vi "Exe1.vi"() -> ()   [LabVIEW 2017]
uses:
  <vilib>/Analysis/4window.llb/windowTd.ctl
  <vilib>/sound2/lvsound2.llb/Sound Data Format.ctl
  <vilib>/sound2/lvsound2.llb/Sampling Mode.ctl
  <extravilib>/ChannelInstances/Stream-a[.](wfm(dbl))/Read With Abort.vi
  <extravilib>/ChannelInstances/Stream-a[.](wfm(dbl))/Write With Abort.vi
  <extravilib>/ChannelInstances/Stream-a[.](wfm(dbl))/EndpointRead.vi
  <extravilib>/ChannelInstances/Stream-a[.](wfm(dbl))/Endpoint.vi
  <extravilib>/ChannelInstances/Stream-a[.](wfm(dbl))/Instantiate.vi
  <extravilib>/ChannelInstances/Stream-a[.](wfm(dbl))/)Channel.vi
  <resource>/ChannelSupport/_ChannelSupport/WaitIfNeeded.vi
  <vilib>/Waveform/WDTFileIO.llb/Export Waveforms To Spreadsheet File (1D).vi
  <vilib>/measure/maspectr.llb/FFT Power Spectrum and PSD for N Chan.vi
  <vilib>/sound2/lvsound2.llb/Sound Input Read (DBL).vi
  <extravilib>/ChannelInstances/Stream-a[.](wfm(dbl)).lvlib
  <vilib>/measure/NI_MAPro.lvlib
  <vilib>/Analysis/NI_AALPro.lvlib
panel:
  in  "file path":path=path "C:/Polimi/2020-data-acquisition-systems/04-ExamPreparation/data.txt"
  out "Acquired Audio PSD":cluster{"f0":dbl, "df":dbl, "magnitude":dbl[]}[](graph)
  in  "dB On (F)":bool
  in  "window":T1=1 items=["Rectangle"=0, "Hanning"=1, "Hamming"=2, "Blackman-Harris"=3, "Exact Blackman"=4, "Blackman"=5, "Flat Top"=6, "4 Term B-Harris "=7, "7 Term B-Harris"=8, "Low Sidelobe"=9, "Blackman Nuttall"=11, "Triangle"=30, "Bartlett-Hanning"=31, "Bohman"=32, "Parzen"=33, "Welch"=34, "Kaiser"=60, "Dolph-Chebyshev"=61, "Gaussian"=62]
  out "Positive Peak":dbl
  out "Negative Peak":dbl
  out "Mean (DC)":dbl
  out "Acquired Audio":waveform(dbl)[](graph)
  in  "stop":bool
  # "Exercise 1"
  # "Exercise 2"
  # "Exercise 3"
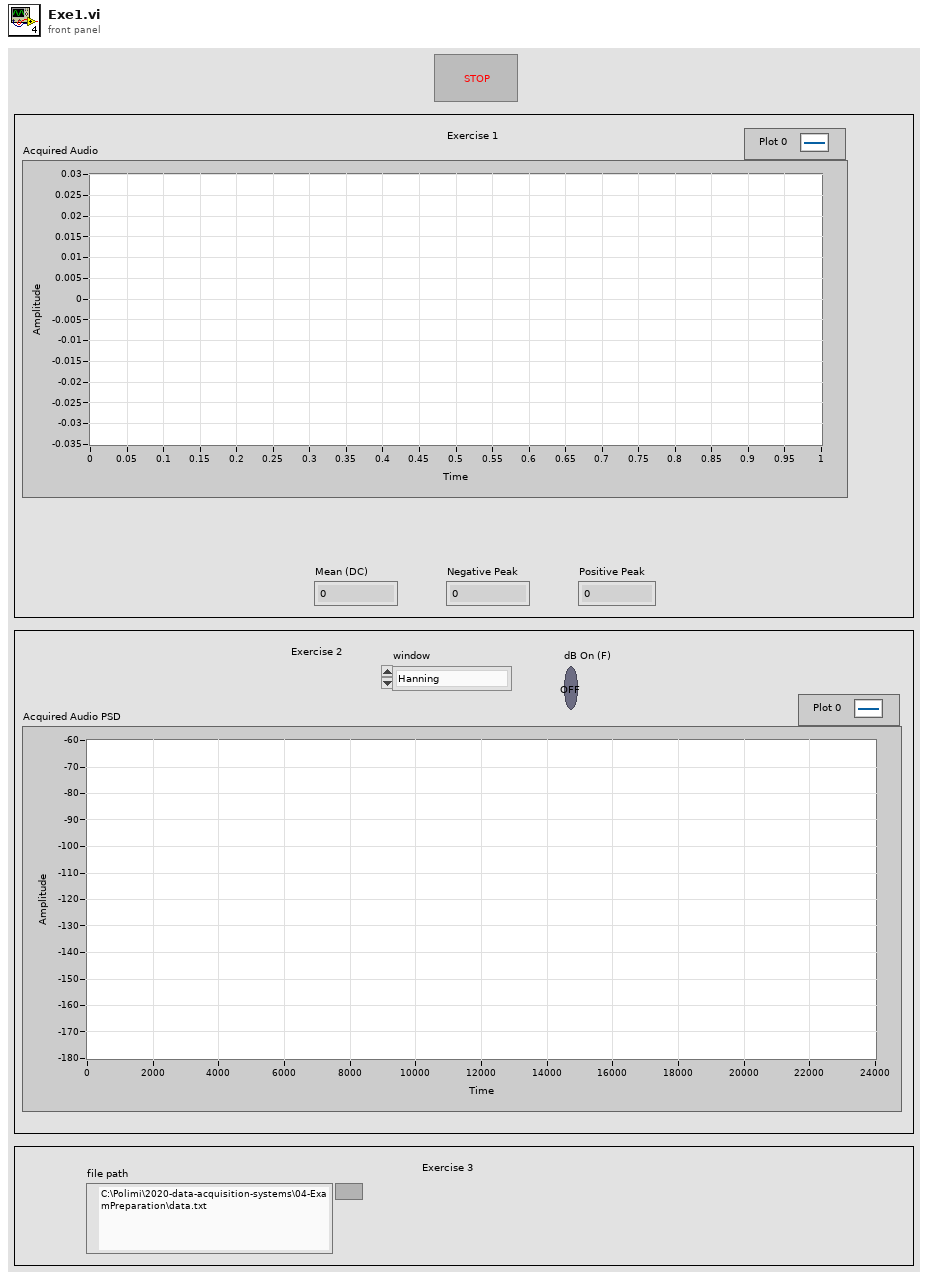
[diagram p1: front panel]
types:
  T1 = typedef "NI_AALPro.lvlib/windowTd.ctl" = u32
  T2 = typedef "Sampling Mode.ctl" = i32
  T3 = typedef "Sound Data Format.ctl" = cluster{"sample rate (S/s)":dbl, "number of channels":i32, "bits per sample":i32}
  T4 = typedef "Sound Input Task ID.ctl" = u32
  T5 = typedef "Stream-a[.](wfm(dbl)).lvlib/)Channel.ctl" = refnum<queue>
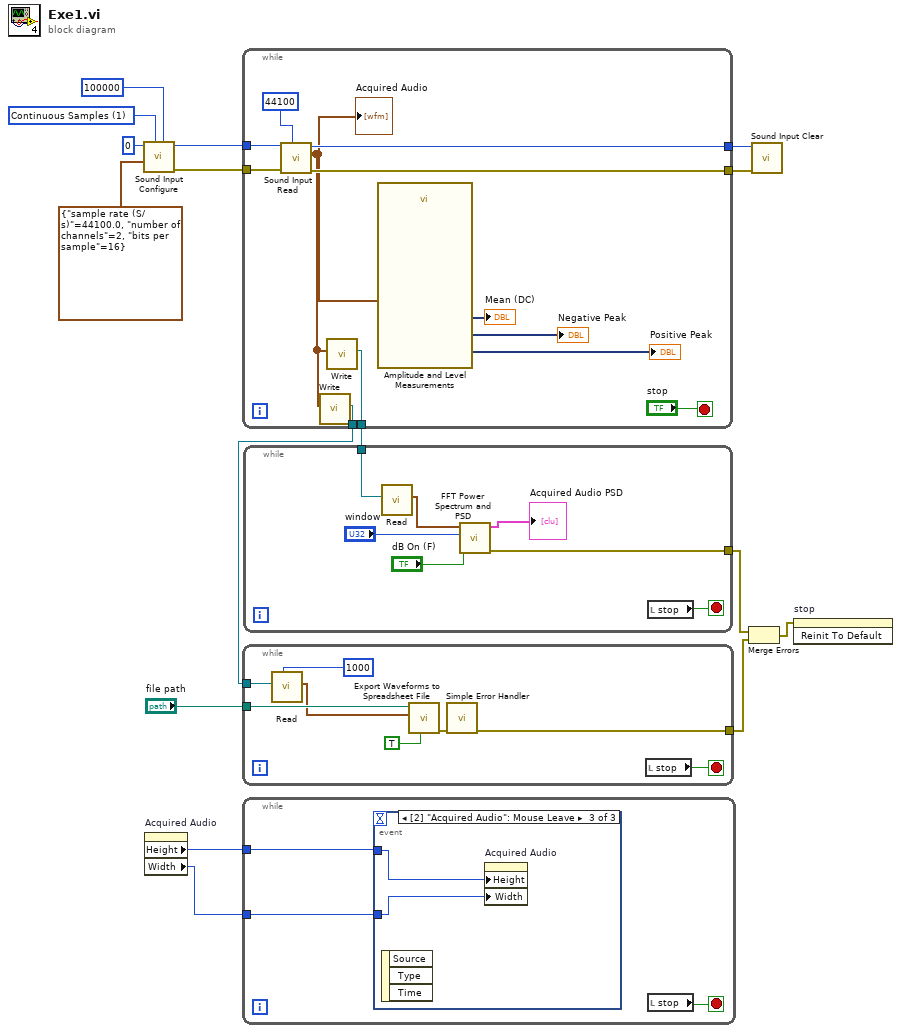
[diagram p0: block diagram]
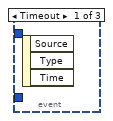
[diagram p2: hidden frame]
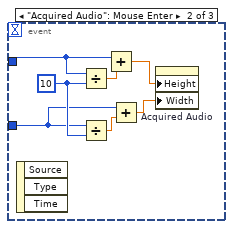
[diagram p3: hidden frame]
diagram:
  w14 = T2 1 items=["Finite Samples", "Continuous Samples"] ("sample mode")
  n1 = call <vilib>:"Sound Input Configure.vi"("number of samples/ch"=100000, "sample mode"=w14, "sound format"=T3 {"sample rate (S/s)"=44100.0, "number of channels"=2, "bits per sample"=16}, "device ID"=u32 0) -> ("error out"=w12:errorcluster, "task ID"=w11:T4)  [unwired: 6 in]
  n2 = property on="Acquired Audio" class="WFGraph (strict)"() -> ("Height"=w2:u32, "Width"=w1:u32)  [unwired: 2 in, 2 out]
  n3 = while {
    tunnel: w12 -> [w27]
    tunnel: w11 -> [w26]
    tunnel: [w25] -> w10
    tunnel: [w24] -> w9
    tunnel: [w18] -> w8
    tunnel: [w17] -> w7
    stop <- "stop" stop-if-true
    n4 = call-poly <vilib>:"Sound Input Read.vi"("number of samples/ch"=44100, "error in (no error)"=w27, "task ID"=w26) -> ("error out"=w24:errorcluster, "data"=w22:waveform(dbl)[], "task ID out"=w25:T4)  [unwired: 6 in]
    "Acquired Audio" <- w22
    n5 = call <extravilib>:"Write.vi"("element"=w22) -> ("channel"=w17:T5)  [unwired: 8 in, 2 out]
    n6 = call <extravilib>:"Write.vi"("element"=w22) -> ("channel"=w18:T5)  [unwired: 8 in, 2 out]
    n7 = call "Amplitude and Level Measurements"("Signals"=w22) -> ("Mean (DC)"=→"Mean (DC)":dynamicdata, "Negative Peak"=→"Negative Peak":dynamicdata, "Positive Peak"=→"Positive Peak":dynamicdata)  [unwired: 11 in, 1 out]
  }
  n8 = while {
    tunnel: w7 -> [w35]
    tunnel: "file path" -> [w33]
    tunnel: [w30] -> w3
    stop <- w36 stop-if-true
    n9 = call <extravilib>:"Read.vi"("timeout in ms (-1)"=1000, "channel"=w35) -> ("element"=w32:waveform(dbl)[])  [unwired: 5 in, 4 out]
    n10 = call-poly <vilib>:"Export Waveforms to Spreadsheet File.vi"("append to file? (new file:F)"=TRUE, "waveforms"=w32, "file path (dialog if empty)"=w33) -> ("error out"=w31:errorcluster)  [unwired: 7 in, 1 out]
    n11 = call <vilib>:"Simple Error Handler.vi"("error in (no error)"=w31) -> ("error out"=w30:errorcluster)  [unwired: 4 in, 4 out]
    n12 = local read "stop"() -> (w36:bool)
  }
  n13 = while {
    tunnel: w2 -> [w38]
    tunnel: w1 -> [w37]
    stop <- w39 stop-if-true
    n14 = event shown="[2] \"Acquired Audio\": Mouse Leave" {
      selector: _ -> [_ _ _]
      dyn-events: _ -> [_ _ _]
      timeout: _ -> [_ _ _]
      tunnel: w38 -> [_ w46 w48]
      tunnel: w37 -> [_ w41 w47]
      event Timeout {
        n15 = event-data() -> ()  [unwired: 1 in, 3 out]
      }
      event "Acquired Audio": Mouse Enter {
        w43 = u32 10 ("y")
        n16 = event-data() -> ()  [unwired: 1 in, 3 out]
        n17 = Divide(x=w46, y=w43) -> (x/y=w45:dbl)
        n18 = Divide(x=w41, y=w43) -> (x/y=w42:dbl)
        n19 = Add(x=w46, y=w45) -> (x+y=w44:dbl)
        n20 = Add(x=w41, y=w42) -> (x+y=w40:dbl)
        n21 = property on="Acquired Audio" class="WFGraph (strict)"("Height"=w44, "Width"=w40) -> ()  [unwired: 2 in, 2 out]
      }
      event "Acquired Audio": Mouse Leave {
        n22 = event-data() -> ()  [unwired: 1 in, 3 out]
        n23 = property on="Acquired Audio" class="WFGraph (strict)"("Height"=w48, "Width"=w47) -> ()  [unwired: 2 in, 2 out]
      }
    }
    n24 = local read "stop"() -> (w39:bool)
  }
  n25 = while {
    tunnel: w8 -> [w55]
    tunnel: [w50] -> w5
    stop <- w51 stop-if-true
    n26 = call <extravilib>:"Read.vi"("channel"=w55) -> ("element"=w54:waveform(dbl)[])  [unwired: 6 in, 4 out]
    n27 = call-poly <vilib>:"FFT Power Spectrum and PSD.vi"("dB On (F)"="dB On (F)", "window"="window", "time signals"=w54) -> ("error out"=w50:errorcluster, "Power Spectrum / PSD"=→"Acquired Audio PSD":cluster{"f0":dbl, "df":dbl, "magnitude":dbl[]}[])  [unwired: 5 in, 2 out]
    n28 = local read "stop"() -> (w51:bool)
  }
  n29 = Merge Errors(w5, w3) -> (w6:errorcluster)
  n30 = call <vilib>:"Sound Input Clear.vi"("error in (no error)"=w9, "task ID"=w10) -> ()  [unwired: 9 in, 1 out]
  n31 = invoke on="stop" class="Bool (strict)" method="Reinit To Default"(error in=w6) -> ()  [unwired: 2 in, 3 out]
